vi "scripting_build_FXP_VIs.vi"() -> ()   [LabVIEW 2020]
uses:
  <vilib>/numeric/LVNumericRepresentation.ctl
panel:
  out "error out 2":errorcluster
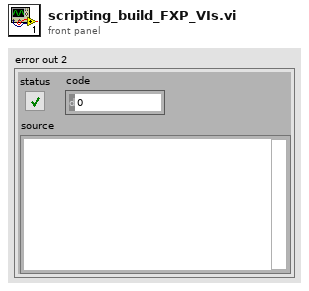
[diagram p1: front panel]
types:
  T1 = typedef "LVNumericRepresentation.ctl" = enum32{"Extended Precision", "Double Precision", "Single Precision", "Long", "Word", "Byte", "Unsigned Long", "Unsigned Word", "Unsigned Byte", "Complex Extended", "Complex Double", "Complex Single", "Quad", "Unsigned Quad", "Fixed-Point"}
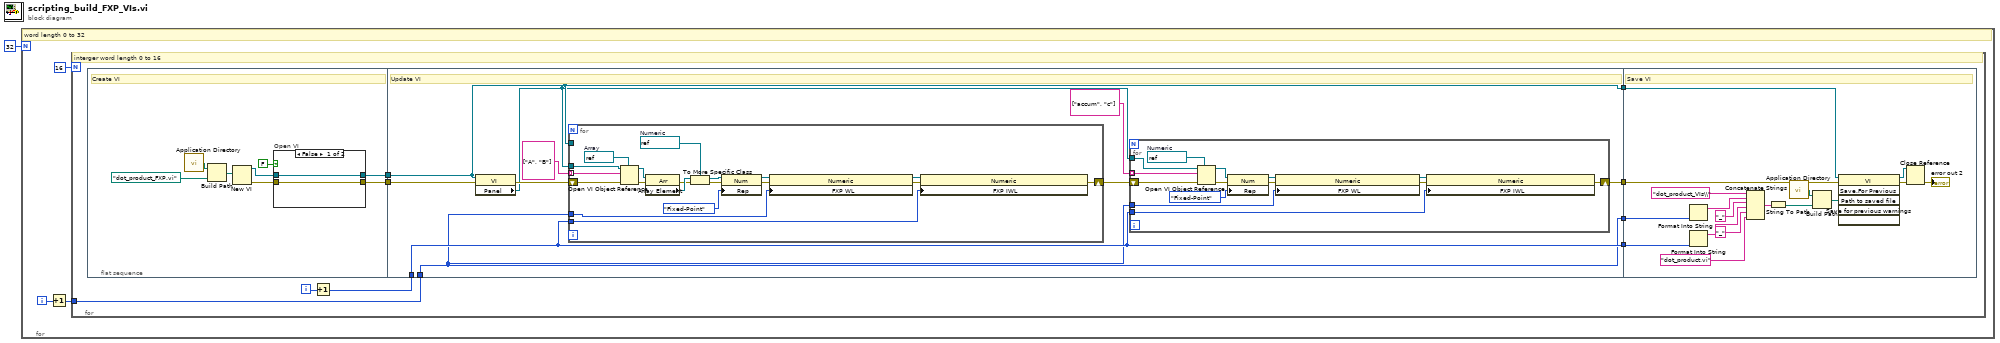
[diagram p0: block diagram]
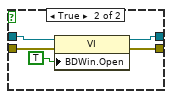
[diagram p2: hidden frame]
diagram:
  n1 = for {
    N: 32 -> [_]
    i -> [w4]
    # "word length 0 to 32"
    n2 = Increment(x=w4) -> (x+1=w2:i32)
    n3 = for {
      N: 16 -> [_]
      tunnel: w2 -> [w7]
      i -> [w6]
      # "interger word length 0 to 16"
      n4 = flat-sequence {
        tunnel: [w14] -> w13
        tunnel: [w15] -> w12
        tunnel: w5 -> [w32]
        tunnel: w7 -> [w31]
        tunnel: w13 -> [w34]
        tunnel: w12 -> [w36]
        tunnel: [w35] -> w11
        tunnel: [w31] -> w10
        tunnel: [w32] -> w9
        tunnel: [w34] -> w8
        tunnel: w11 -> [w76]
        tunnel: w10 -> [w72]
        tunnel: w9 -> [w73]
        tunnel: w8 -> [w74]
        frame #0 {
          # "Create VI"
          n5 = call <vilib>:"Application Directory.vi"() -> ("Application Directory"=w20:path)
          n6 = Build Path(base path=w20, name or relative path=path "dot_product_FXP.vi" ("vi path")) -> (appended path=w21:path)
          n7 = New VI(10:w21) -> (0:w19:errorcluster, 3:w18:refnum<vi>)  [unwired: 6 in]
          n8 = case "Open VI" shown="False" FALSE {
            tunnel: w18 -> [w22 w28]
            tunnel: w19 -> [w23 w27]
            tunnel: [w22 w25] -> w14
            tunnel: [w23 w24] -> w15
            frame False {
            }
            frame True {
              n9 = property class="VI"(reference=w28, error in=w27, "BDWin.Open"=TRUE ("Block Diagram Window:Open")) -> (reference out=w25:refnum<vi>, error out=w24:errorcluster)
            }
          }
        }
        frame #1 {
          # "Update VI"
          n10 = property on="Property Node" class="VI"(reference=w34, error in=w36) -> (error out=w38:errorcluster, "Panel"=w30:refnum<vi>)  [unwired: 1 out]
          n11 = for {
            tunnel: w30 -> [w68]
            shift-right: [w56] -> w29
            shift-left: w38 -> [w70]
            tunnel: string[] ["A", "B"] -> [w69] mode=indexing
            tunnel: w34 -> [_]
            tunnel: w31 -> [w54]
            tunnel: w32 -> [w53]
            w66 = refnum<vi> refnum  # Numeric
            w71 = refnum<vi> refnum  # Array
            n12 = Open VI Object Reference(7:w71, 8:w70, 10:w69, 11:w68) -> (0:w62:errorcluster, 3:w63:refnum<vi>)
            n13 = property class="Arr"(reference=w63, error in=w62) -> (error out=w61:errorcluster, "Array Element"=w67:refnum<vi>)  [unwired: 1 out]
            n14 = To More Specific Class(target class=w66, reference=w67, error in=w61) -> (specific class reference=w65:refnum<vi>, error out=w60:errorcluster)
            n15 = property class="Num"(reference=w65, error in=w60, "Rep"=LVNumericRepresentation."Fixed-Point" ("Representation")) -> (reference out=w59:refnum<vi>, error out=w55:errorcluster)
            n16 = property on="Property Node" class="Numeric"(reference=w59, error in=w55, "FXP WL"=w54) -> (reference out=w58:refnum<vi>, error out=w57:errorcluster)
            n17 = property on="Property Node" class="Numeric"(reference=w58, error in=w57, "FXP IWL"=w53) -> (error out=w56:errorcluster)  [unwired: 1 out]
          }
          n18 = for {
            tunnel: w30 -> [w48]
            shift-right: [w41] -> w35
            shift-left: w29 -> [w51]
            tunnel: string[] ["accum", "c"] -> [w46] mode=indexing
            tunnel: w31 -> [w40]
            tunnel: w32 -> [w39]
            w52 = refnum<vi> refnum  # Numeric
            n19 = Open VI Object Reference(7:w52, 8:w51, 10:w46, 11:w48) -> (0:w49:errorcluster, 3:w50:refnum<vi>)
            n20 = property class="Num"(reference=w50, error in=w49, "Rep"=LVNumericRepresentation."Fixed-Point" ("Representation")) -> (reference out=w43:refnum<vi>, error out=w42:errorcluster)
            n21 = property on="Property Node" class="Numeric"(reference=w43, error in=w42, "FXP WL"=w40) -> (reference out=w45:refnum<vi>, error out=w44:errorcluster)
            n22 = property on="Property Node" class="Numeric"(reference=w45, error in=w44, "FXP IWL"=w39) -> (error out=w41:errorcluster)  [unwired: 1 out]
          }
        }
        frame #2 {
          # "Save VI"
          n23 = Format Into String(w72) -> (resulting string=w86:string)  [unwired: 3 in, 1 out]
          n24 = Format Into String(w73) -> (resulting string=w87:string)  [unwired: 3 in, 1 out]
          n25 = Concatenate Strings("dot_product_VIs\\" ("string"), w86, "_" ("string"), w87, "_" ("string"), "dot_product.vi" ("string")) -> (w75:string)
          n26 = String To Path(string=w75) -> (path=w88:path)
          n27 = call <vilib>:"Application Directory.vi"() -> ("Application Directory"=w84:path)
          n28 = Build Path(base path=w84, name or relative path=w88) -> (appended path=w85:path)
          n29 = invoke class="VI" method="Save.For Previous"(reference=w74, error in=w76, "Path to saved file"=w85) -> (reference out=w81:refnum<vi>, error out=w82:errorcluster)  [unwired: 3 in, 4 out]
          n30 = Close Reference(reference=w81, error in (no error)=w82) -> (error out=→"error out 2":errorcluster)
        }
      }
      n31 = Increment(x=w6) -> (x+1=w5:i32)
    }
  }
